vi "TransformacionPatron.vi"(2 "Patrón original":T1, 3 "Toma original":T1) -> (0 "Patron Original":T1(plugin-control) caption="Perfil lateral", 1 "Toma corregida":T1(plugin-control) caption="Perfil lateral")   [LabVIEW 2021]
doc: "Traslada el patrón a la misma posición que la toma de la cámara para empalmar sus contornos"
uses:
  <vilib>/vision/Image Controls.llb/IMAQ Image.ctl
panel:
  out "Centroide Patron":cluster{"X Centroid":sgl, "Y Centroid":sgl}
  out "Centroide Captura":cluster{"X Centroid":sgl, "Y Centroid":sgl}
  # "CUEVAS CERÓN SERGIO ALBERTO\nREYES PÉREZ JAVIER\nSALCEDO LICEA JUAN CARLOS"
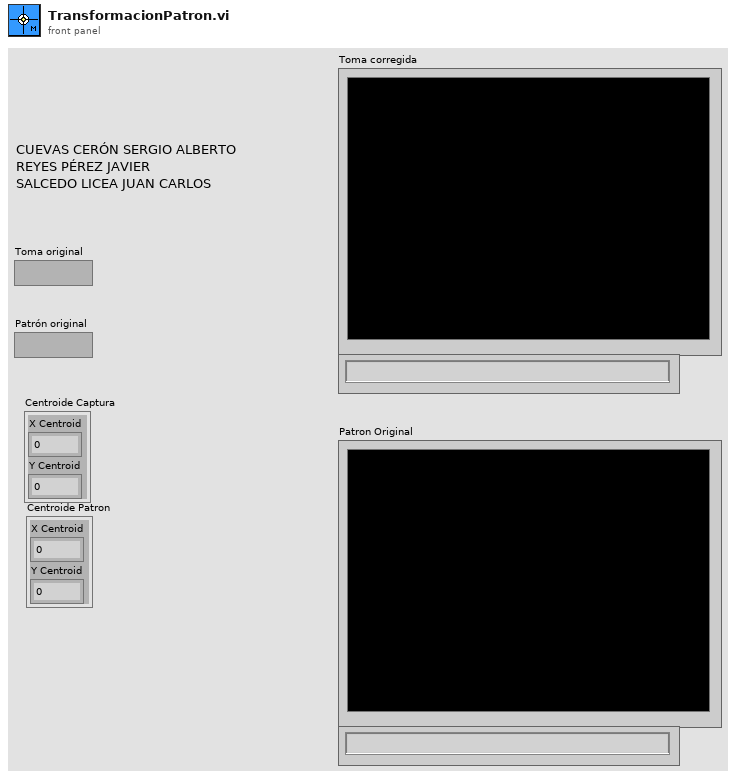
[diagram p1: front panel]
types:
  T1 = typedef "IMAQ Image.ctl" = refnum<image>
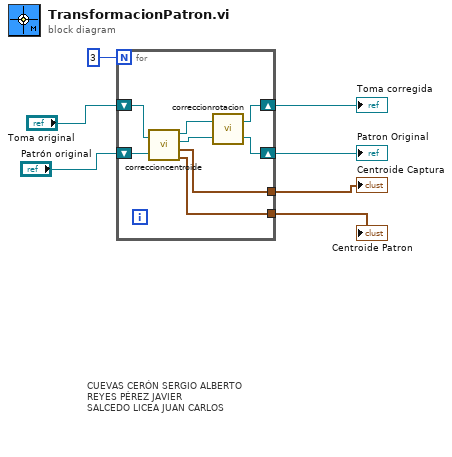
[diagram p0: block diagram]
diagram:
  # "CUEVAS CERÓN SERGIO ALBERTO\nREYES PÉREZ JAVIER\nSALCEDO LICEA JUAN CARLOS"
  n1 = for {
    N: 3 -> [_]
    shift-right: [w10] -> w4
    shift-left: "Patrón original" -> [w13]
    shift-right: [w11] -> w5
    shift-left: "Toma original" -> [w12]
    tunnel: [w9] -> w2
    tunnel: [w8] -> w1
    n2 = call "correccioncentroide.vi"("Toma Original"=w12, "Patrón original"=w13) -> ("Tom trasladada"=w14:T1, "Patron original(dup)"=w15:T1, "Centroide Captura"=w9:cluster{"X Centroid":sgl, "Y Centroid":sgl}, "Centroide Patron"=w8:cluster{"X Centroid":sgl, "Y Centroid":sgl})
    n3 = call "correccionrotacion.vi"("Patron original"=w15, "Toma original"=w14) -> ("Patron original (dupl)"=w10:T1, "Toma rotada"=w11:T1)
  }
  "Toma corregida" <- w5
  "Patron Original" <- w4
  "Centroide Captura" <- w2
  "Centroide Patron" <- w1
